vi "CLC_JIO_subBFIC_disable.vi"(8 "error in":errorcluster) -> (0 "error out":errorcluster, 3 "standard output":string)   [LabVIEW 2023, in "CLC_JIO_FTDI.lvlib"]
uses:
  CLC_JIO_FTDI.lvlib
panel:
  out "resulting string":string
  out "appended path":path
  out "standard error":string
  out "Check driver floder?":bool
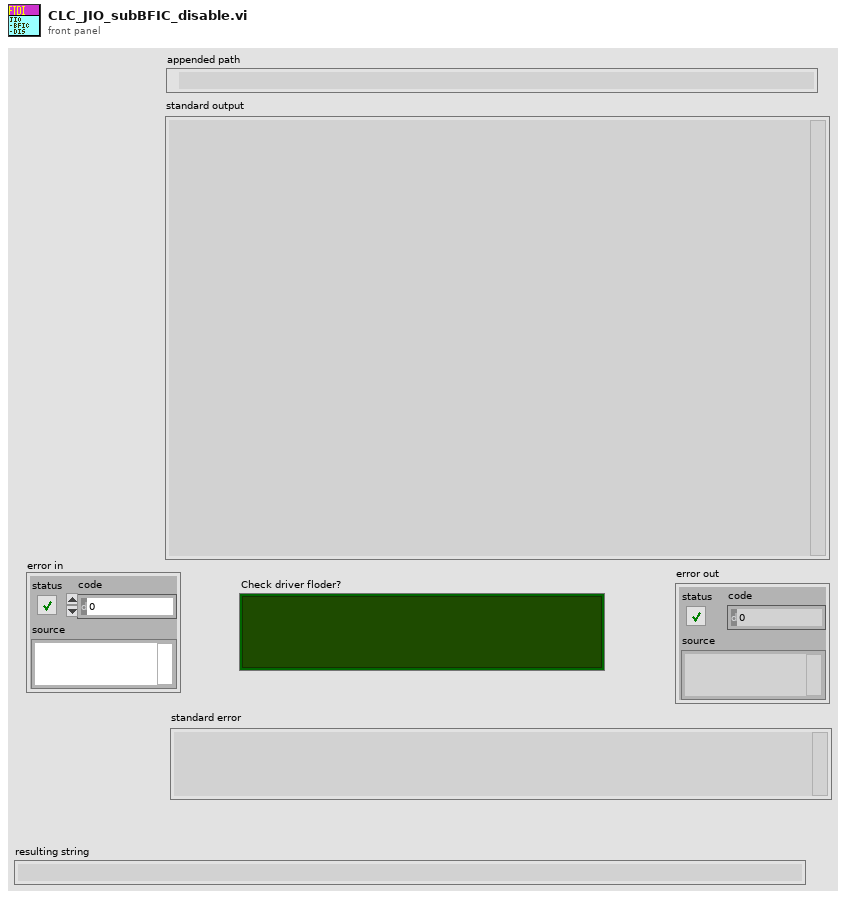
[diagram p1: front panel]
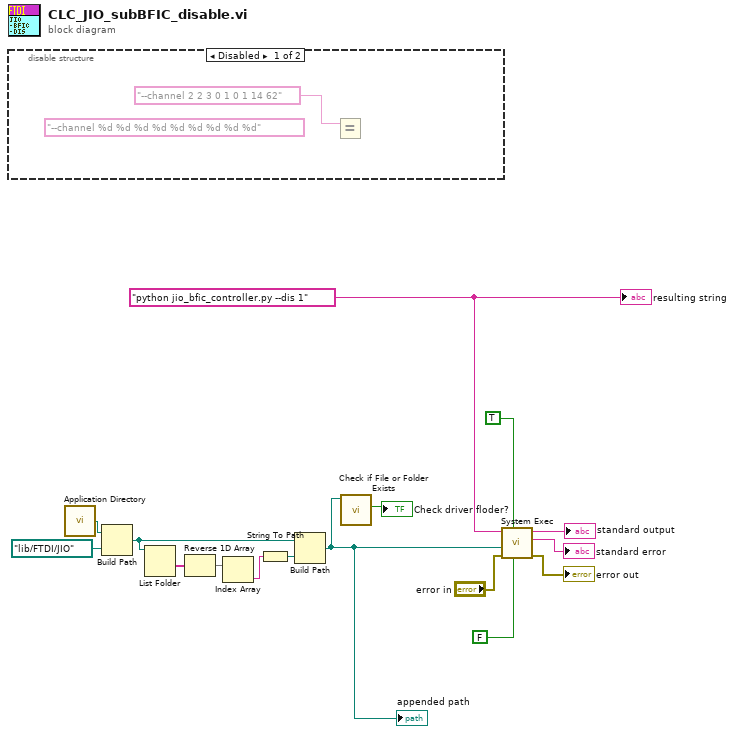
[diagram p0: block diagram]
diagram:
  w1 = "python jio_bfic_controller.py --dis 1" ("command line")
  n1 = disable-structure shown="Disabled" {
    frame Disabled {
      (unwired) "--channel %d %d %d %d %d %d %d %d %d" ("command line")
      n2 = Equal?(x="--channel 2 2 3 0 1 0 1 14 62") -> ()  [unwired: 1 in, 1 out]
    }
    frame Enabled {
    }
  }
  n3 = call <vilib>:"Application Directory.vi"() -> ("Application Directory"=w10:path)
  n4 = Build Path(base path=w10, name or relative path=path "lib/FTDI/JIO") -> (appended path=w9:path)
  n5 = List Folder(path=w9) -> (folder names=w15:string[])  [unwired: 3 in, 3 out]
  n6 = Reverse 1D Array(array=w15) -> (reversed array=w14:string[])
  n7 = Index Array(array=w14) -> (element=w13:string)  [unwired: 1 in]
  n8 = String To Path(string=w13) -> (path=w12:path)
  n9 = Build Path(base path=w9, name or relative path=w12) -> (appended path=w7:path)
  "appended path" <- w7
  n10 = call <vilib>:"Check if File or Folder Exists.vi"("path"=w7) -> ("file or folder exists?"=→"Check driver floder?":bool)  [unwired: 8 in, 2 out]
  n11 = call <vilib>:"System Exec.vi"("run minimized? (F)"=FALSE, "wait until completion? (T)"=TRUE, "error in (no error)"="error in", "working directory"=w7, "command line"=w1) -> ("error out"=→"error out":errorcluster, "standard error"=→"standard error":string, "standard output"=→"standard output":string)  [unwired: 3 in, 1 out]
  "resulting string" <- w1
